vi "GT Compare Linear.vi"(0 "cardNum":i16, 1 "repeatTimes":i32, 2 "time":i16, 5 "encoder":i16, 7 "channel":i16, 9 "startPos":i32, 11 "error in (no error)":errorcluster caption="错误输入（无错误）", 12 "interval":i32, 13 "source":i16) -> (4 "function return":i16, 15 "error out":errorcluster caption="错误输出")   [LabVIEW 2020, in "gts.lvlib"]
doc: "GT_API GT_CompareLinear(short cardNum,short encoder,short channel,long startPos,long repeatTimes,long interval,short time,short source);"
uses:
  gts.lvlib
  dll/32bit/multi_card/gts.dll
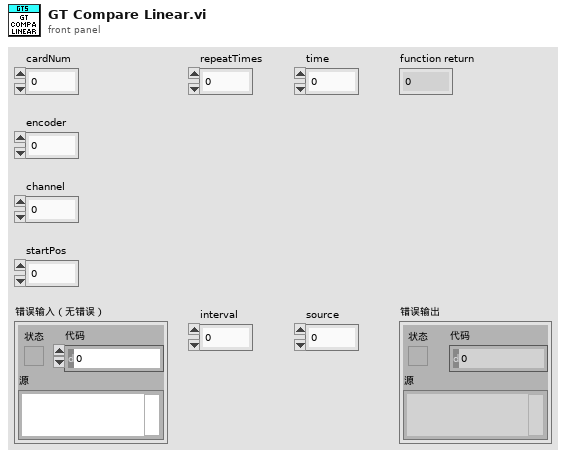
[diagram p1: front panel]
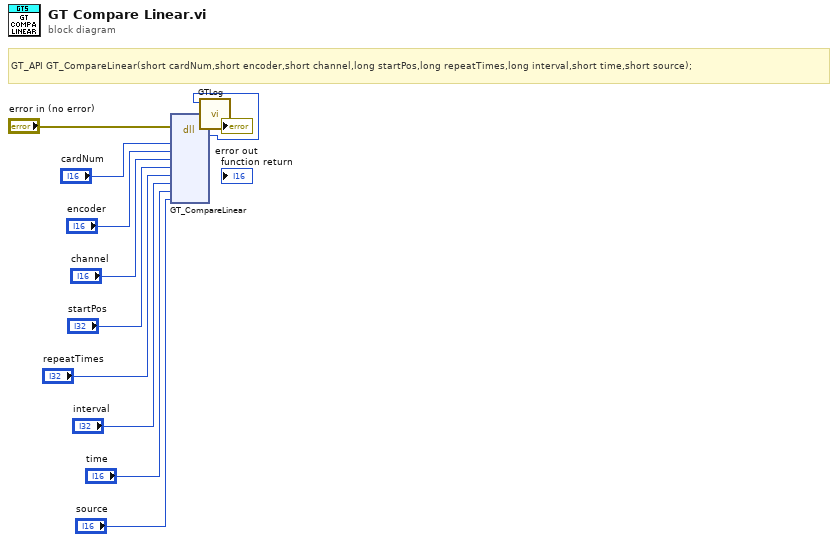
[diagram p0: block diagram]
diagram:
  # "GT_API GT_CompareLinear(short cardNum,short encoder,short channel,long startPos,long repeatTimes,long interval,short time,short source);"
  n1 = dll-call lib="C:/1228/dll/32bit/multi_card/gts.dll" fn="GT_CompareLinear"(error in="error in (no error)", "cardNum"="cardNum", "encoder"="encoder", "channel"="channel", "startPos"="startPos", "repeatTimes"="repeatTimes", "interval"="interval", "time"="time", "source"="source") -> (error out=w3:errorcluster, w1:i16)  [unwired: 10 in, 1 out]
  n2 = call "GTLog.vi"("error in (no error)"=w3, "Numeric"=w1) -> ("error out"=→"error out":errorcluster)  [unwired: 9 in]
